vi "Ex6 Color Thershold.vi"() -> ()   [LabVIEW 2020]
panel:
  in  "Color Mode (Color Threshold 1)":u16(ring)=2 items=["RGB", "HSL", "HSV", "HSI"]
  in  "Blue or Val  (Color Threshold 1)":cluster{"Lower value":i32, "Upper value":i32}={"Lower value"=5, "Upper value"=255}
  in  "Green or Sat Range (Color Threshold 1)":cluster{"Lower value":i32, "Upper value":i32}={"Lower value"=0, "Upper value"=255}
  in  "Red or Hue Range (Color Threshold 1)":cluster{"Lower value":i32, "Upper value":i32}={"Lower value"=28, "Upper value"=90}
  out "error out":errorcluster
  out "Color Channel":T1(plugin-control)
  out "Image":T1(plugin-control)
  in  "File Path":path
  # "EX.6 COLOR THRESHOLD"
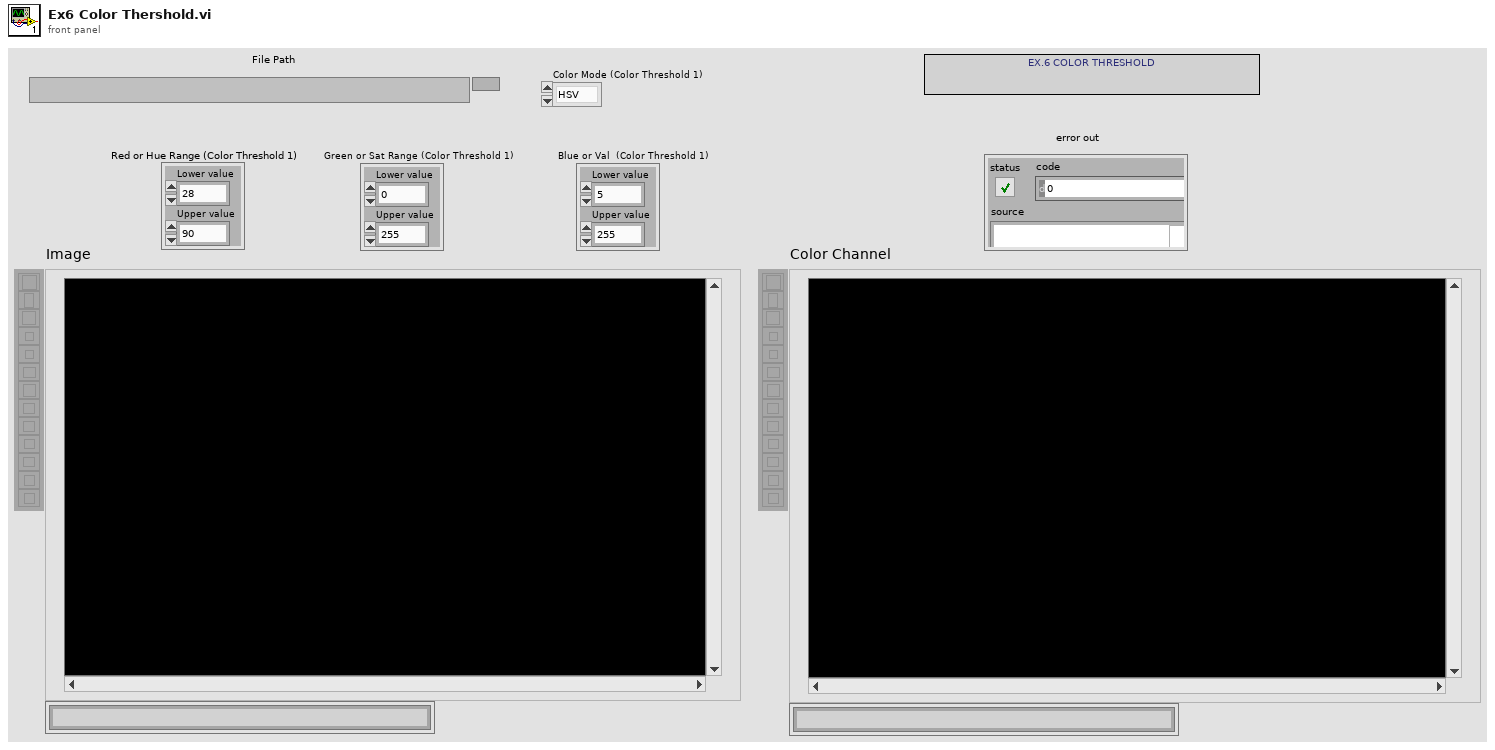
[diagram p1: front panel]
types:
  T1 = typedef "IMAQ Image.ctl" = refnum<image>
  T2 = typedef "Image Type" = u32
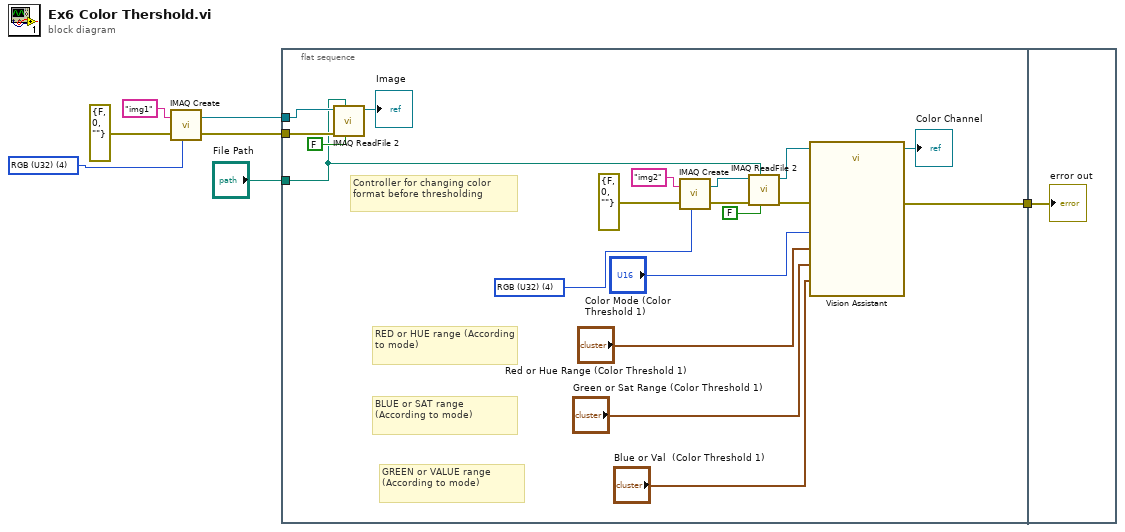
[diagram p0: block diagram]
diagram:
  w1 = T2 4 items=["Grayscale (U8)", "Grayscale (I16)", "Grayscale (SGL)", "Complex (CSG)", "RGB (U32)", "HSL (U32)", "RGB (U64)", "Grayscale (U16)"] ("Image Type")
  n1 = call "IMAQ Create"("Image Name"="img1", "Image Type"=w1, "error in (no error)"=errorcluster {"status"=FALSE, "code"=0, "source"=""}) -> ("New Image"=w2:T1, "error out"=w3:errorcluster)  [unwired: 2 in]
  n2 = flat-sequence {
    tunnel: "File Path" -> [w15]
    tunnel: w3 -> [w25]
    tunnel: w2 -> [w24]
    tunnel: [w22] -> w7
    tunnel: w7 -> [w27]
    frame #0 {
      w19 = T2 4 items=["Grayscale (U8)", "Grayscale (I16)", "Grayscale (SGL)", "Complex (CSG)", "RGB (U32)", "HSL (U32)", "RGB (U64)", "Grayscale (U16)"] ("Image Type")
      # "GREEN or VALUE range (According to mode)"
      # "BLUE or SAT range (According to mode)"
      # "RED or HUE range (According to mode)"
      # "Controller for changing color format before thresholding"
      n3 = call "IMAQ ReadFile 2"("Use File Path Image Type"=FALSE, "File Path"=w15, "error in (no error)"=w25, "Image"=w24) -> ("Image Out"=→"Image":T1)  [unwired: 3 in, 4 out]
      n4 = call "IMAQ Create"("Image Name"="img2", "Image Type"=w19, "error in (no error)"=errorcluster {"status"=FALSE, "code"=0, "source"=""}) -> ("New Image"=w18:T1, "error out"=w17:errorcluster)  [unwired: 2 in]
      n5 = call "IMAQ ReadFile 2"("Use File Path Image Type"=FALSE, "File Path"=w15, "error in (no error)"=w17, "Image"=w18) -> ("error out"=w13:errorcluster, "Image Out"=w14:T1)  [unwired: 3 in, 3 out]
      n6 = call "Vision Assistant"("Image In"=w14, "Color Mode (Color Threshold 1)"="Color Mode (Color Threshold 1)", "Red or Hue Range (Color Threshold 1)"="Red or Hue Range (Color Threshold 1)", "Green or Sat Range (Color Threshold 1)"="Green or Sat Range (Color Threshold 1)", "Blue or Luma or Val or Inten Range (Color Threshold 1)"="Blue or Val  (Color Threshold 1)", "error in"=w13) -> ("Image Out"=→"Color Channel":T1, "error out"=w22:errorcluster)  [unwired: 20 in]
    }
    frame #1 {
      "error out" <- w27
    }
  }
